vi "zigzag.vi"(4 "angulo":dbl=90.0 format="%#_13g", 6 "points 3":cluster{"x":dbl, "y":dbl}[](array[cluster])=[{"x"=0.0, "y"=0.0}, {"x"=1000.0, "y"=1000.0}, {"x"=-1000.0, "y"=1000.0}], 8 "output angle":dbl=4.0, 9 "output xy":dbl=2.0, 10 "Current Robot":T1={"id"=0, "function"=enum."Attacker", "x"=0.0, "y"=0.0, "orientation"=0.0, "v_tangent"=0.0, "v_normal"=0.0, "v_ang"=0.0, "kick_x"=0.0, "kick_z"=0.0, "dribble"=FALSE, "Timestamp"=timestamp(0 s since 1904-01-01), "dest_x"=0.0, "dest_y"=0.0, "dest_orientation"=0.0, "estimatives"={"est_v_tangent"=0.0, "est_v_normal"=0.0, "est_vx"=0.0, "est_vy"=0.0, "Pos Robot Est"=[]}, "dest_x_kick"=0.0, "dest_y_kick"=0.0, "Gap Coord"=[], "States"=enum."GoToTangent", "Path "=[], "Path  Smooth"=[], "dest_vel"=0.0}, 11 "Al Input":T4={"our_robots"=[], "enemy_robots"=[], "balls"=[], "geometry"={"line_width"=0, "field_length"=0, "field_width"=0, "boundary_width"=0, "referee_width"=0, "goal_width"=0, "goal_depth"=0, "goal_wall_width"=0, "center_circle_radius"=0, "defense_radius"=0, "defense_stretch"=0, "free_kick_from_defense_dist"=0, "penalty_spot_from_field_line_dist"=0, "penalty_line_from_spot_dist"=0}, "IA Judge"={"stage"="", "command"="", "our_goalie_id"=0.0, "enemy_goalie_id"=0.0, "command enum"=enum."Halt", "Time"=enum."Azul"}, "Received Timestamp"=timestamp(0 s since 1904-01-01), "Events"={"Touch"=FALSE, "Ball out"=FALSE, "id touch"=0.0, "Ball out of \nVision"=FALSE, "Ball inside \nGoalie area"=FALSE, "Robot not responding"=FALSE, "Robots responding status"=[1.0, 1.0, 1.0, 1.0, 1.0, 1.0], "Enemy Ball \nPossession"=FALSE, "Pass State"=FALSE, "id end of pass"=0.0, "Kick"=FALSE, "Id ini Possession"=0.0, "Ball Possesion"=FALSE, "Id Possesion"=0.0}}) -> (3 "Output Robot":T1={"id"=0, "function"=enum."Attacker", "x"=0.0, "y"=0.0, "orientation"=0.0, "v_tangent"=0.0, "v_normal"=0.0, "v_ang"=0.0, "kick_x"=0.0, "kick_z"=0.0, "dribble"=FALSE, "Timestamp"=timestamp(0 s since 1904-01-01), "dest_x"=0.0, "dest_y"=0.0, "dest_orientation"=0.0, "estimatives"={"est_v_tangent"=0.0, "est_v_normal"=0.0, "est_vx"=0.0, "est_vy"=0.0, "Pos Robot Est"=[]}, "dest_x_kick"=0.0, "dest_y_kick"=0.0, "Gap Coord"=[], "States"=enum."GoToTangent", "Path "=[], "Path  Smooth"=[], "dest_vel"=0.0})   [LabVIEW 2017]
uses:
  Core/AI Input.ctl
  Core/AI Robot.ctl
  Intel/Functions Enum.ctl
  Intel/AttackerStates.ctl
  Core/AI Ball.ctl
  Core/Field Size.ctl
  Core/AI Judge.ctl
  Intel/Command Enum.ctl
  Util/Events/Events.ctl
panel:
  out "Waveform Chart 3":dbl(graph)
  out "Waveform Chart 2":dbl(graph)
  out "Waveform Chart":dbl(graph)
  in  "polar tolerance":dbl=50.0 format="%#_13g"
  in  "?":bool=TRUE
  out "element 2":cluster{"x":dbl, "y":dbl}
  in  "square tolerance":dbl=50.0 format="%#_13g"
  # "polar check"
  # "cartesian check"
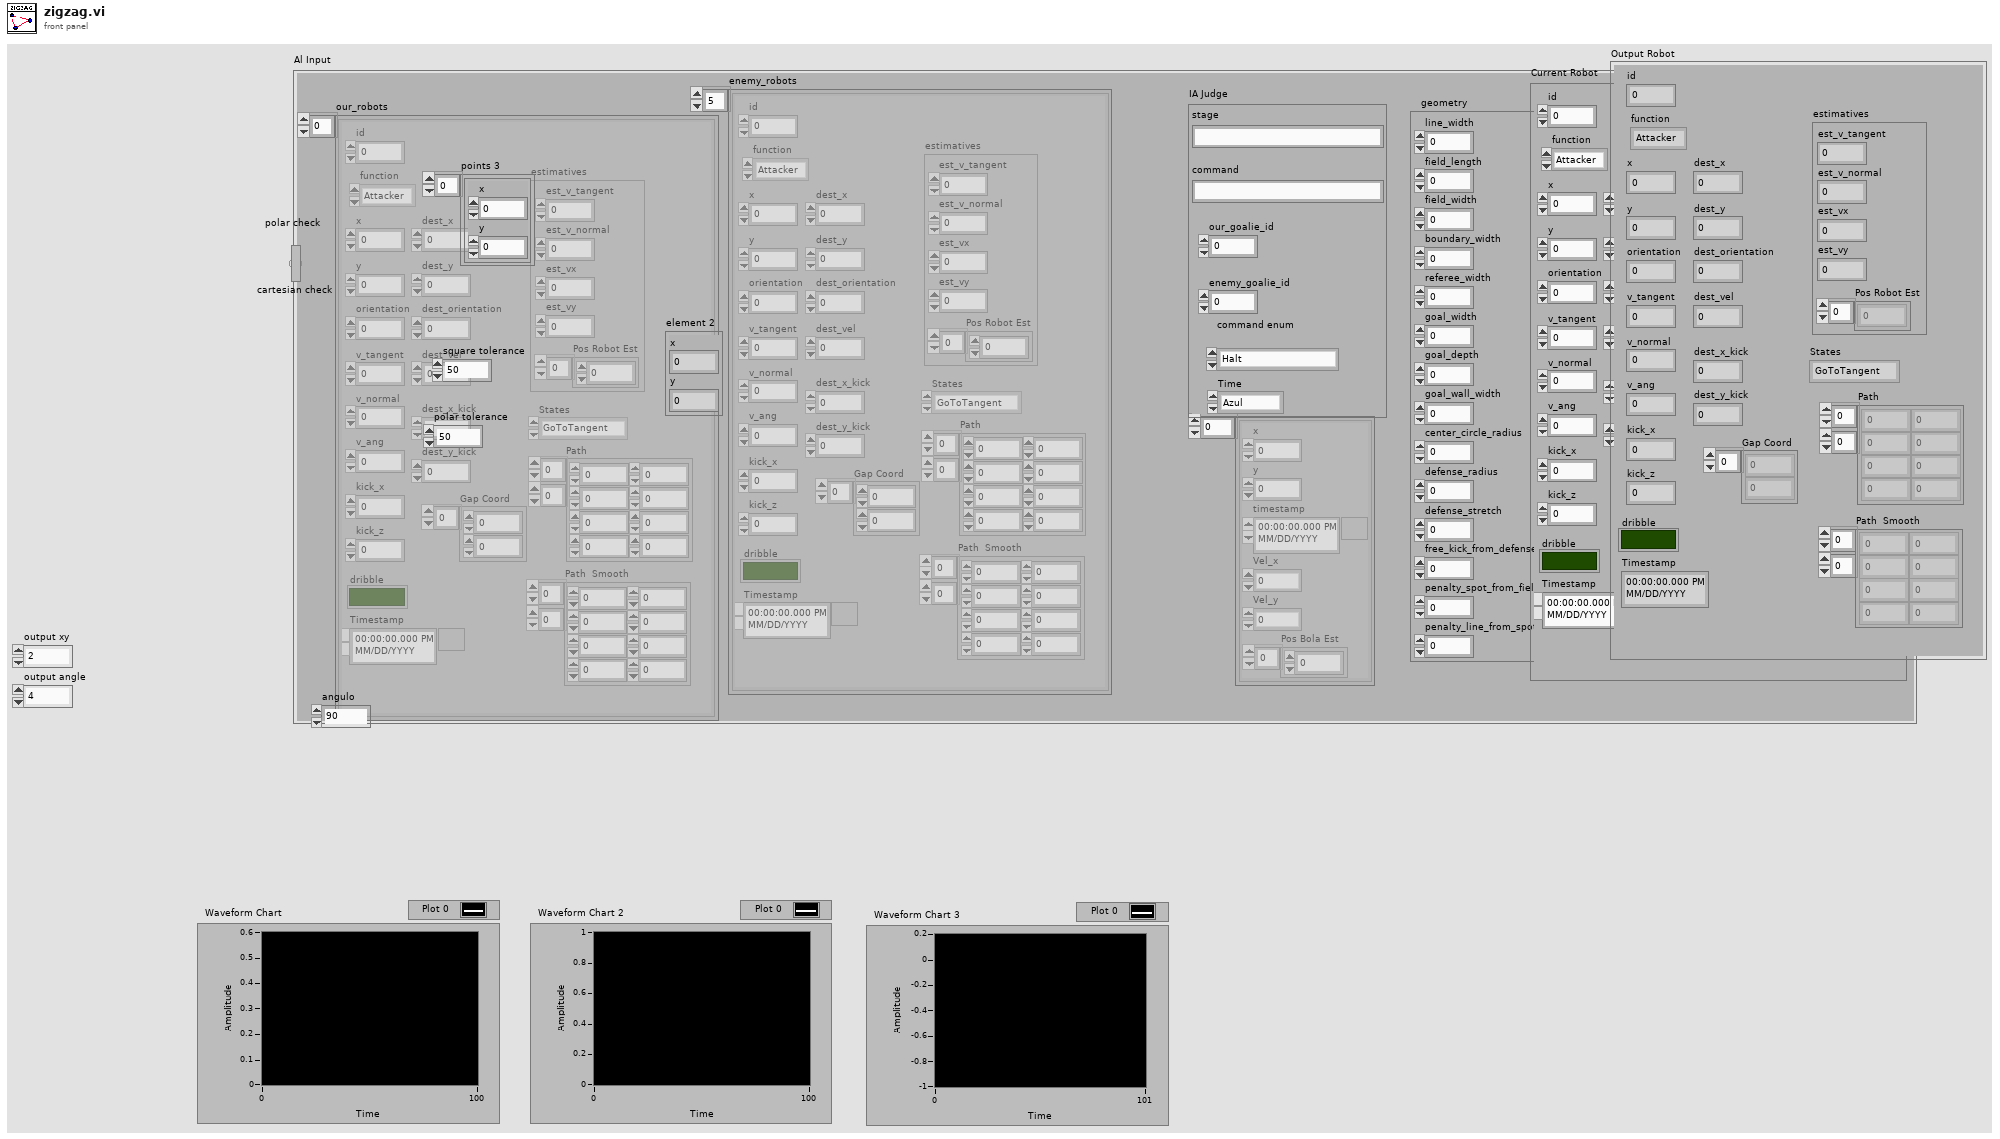
[diagram p1: front panel]
types:
  T1 = typedef "AI Robot.ctl" = cluster{"id":u32, "function":T2, "x":dbl, "y":dbl, "orientation":dbl, "v_tangent":dbl, "v_normal":dbl, "v_ang":dbl, "kick_x":dbl, "kick_z":dbl, "dribble":bool, "Timestamp":timestamp, "dest_x":dbl, "dest_y":dbl, "dest_orientation":dbl, "estimatives":cluster{"est_v_tangent":dbl, "est_v_normal":dbl, "est_vx":dbl, "est_vy":dbl, "Pos Robot Est":dbl[]}, "dest_x_kick":dbl, "dest_y_kick":dbl, "Gap Coord":dbl[], "States":T3, "Path ":dbl[][], "Path  Smooth":dbl[][], "dest_vel":dbl}
  T2 = typedef "Functions Enum.ctl" = enum16{"Attacker", "Goalie", "Defender", "Striker", "Goto 0", "Dummy", "Kicker", "ZigZag"}
  T3 = typedef "AttackerStates.ctl" = enum16{"Pass", "GoToTangent", "BallGetting", "GoToKick", ""}
  T4 = typedef "AI Input.ctl" = cluster{"our_robots":T1[], "enemy_robots":T1[], "balls":T5[], "geometry":T6, "IA Judge":T7, "Received Timestamp":timestamp, "Events":T9}
  T5 = typedef "AI Ball.ctl" = cluster{"x":dbl, "y":dbl, "timestamp":timestamp, "Vel_x":dbl, "Vel_y":dbl, "Pos Bola Est":dbl[]}
  T6 = typedef "Field Size.ctl" = cluster{"line_width":u32, "field_length":u32, "field_width":u32, "boundary_width":u32, "referee_width":u32, "goal_width":u32, "goal_depth":u32, "goal_wall_width":u32, "center_circle_radius":u32, "defense_radius":u32, "defense_stretch":u32, "free_kick_from_defense_dist":u32, "penalty_spot_from_field_line_dist":u32, "penalty_line_from_spot_dist":u32}
  T7 = typedef "AI Judge.ctl" = cluster{"stage":string, "command":string, "our_goalie_id":dbl, "enemy_goalie_id":dbl, "command enum":T8, "Time":enum16{"Azul", "Amarelo"}}
  T8 = typedef "Command Enum.ctl" = enum16{"Halt", "Stop", "Force Start", "PKA Normal Start", "Prepare Kickoff Ally", "PKE Normal Start", "Prepare Kickoff Enemy", "Prepare Penalty Ally", "PPA Normal Start", "Prepare Penalty Enemy", "PPE Normal Start", "Direct Free Enemy", "Direct Free Ally", "Indirect Free Enemy", "Indirect Free Ally", "Timeout Enemy", "Timeout Ally", "Goal Enemy", "Goal Ally", "Ball Placement Enemy", "Ball Placement Ally", "Normal Half Time", "Extra Time Break", "Extra Half Time", "None", "Post Game"}
  T9 = typedef "Events.ctl" = cluster{"Touch":bool, "Ball out":bool, "id touch":dbl, "Ball out of \nVision":bool, "Ball inside \nGoalie area":bool, "Robot not responding":bool, "Robots responding status":dbl[], "Enemy Ball \nPossession":bool, "Pass State":bool, "id end of pass":dbl, "Kick":bool, "Id ini Possession":dbl, "Ball Possesion":bool, "Id Possesion":dbl}
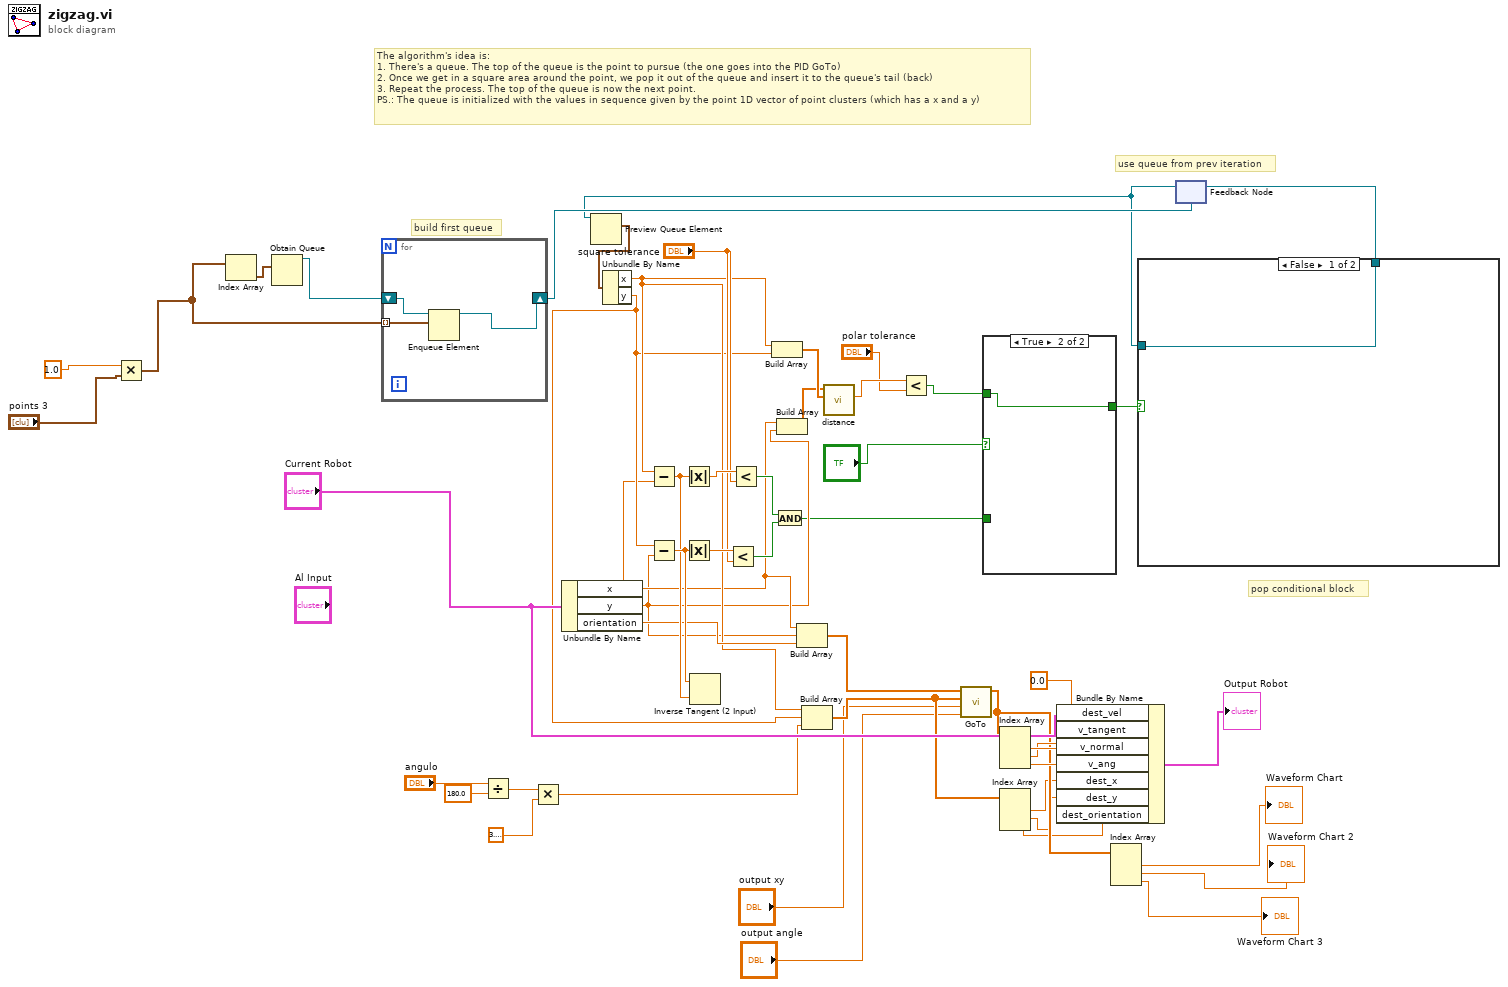
[diagram p0: block diagram]
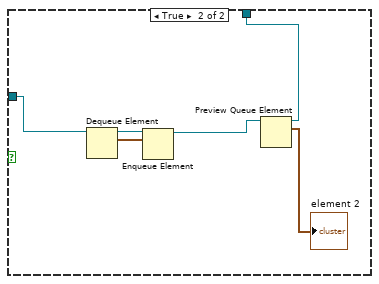
[diagram p3: hidden frame]
diagram:
  # "pop conditional block"
  # "use queue from prev iteration"
  # "The algorithm's idea is:\n1. There's a queue. The top of the queue is the point to pursue (the one goes into the PID GoTo)\n2. Once we get in a square area around the point, we pop it out of the queue and insert it to the queue's tail (back)\n3. Repeat the process. The top of the queue is now the next point.\nPS.: The queue is initialized with the values in sequence given by the point 1D vector of point clusters (which has a x and a y)"
  # "build first queue"
  n1 = Multiply(x=1.0, y="points 3") -> (x*y=w17:cluster{"x":dbl, "y":dbl}[])
  n2 = Index Array(array=w17) -> (element=w51:cluster{"x":dbl, "y":dbl})  [unwired: 1 in]
  n3 = Obtain Queue(element data type=w51) -> (queue out=w50:refnum<queue>)  [unwired: 4 in, 2 out]
  n4 = for {
    tunnel: w17 -> [w53] mode=indexing
    shift-right: [w54] -> w43
    shift-left: w50 -> [w52]
    n5 = Enqueue Element(queue=w52, element=w53) -> (queue out=w54:refnum<queue>)  [unwired: 2 in, 2 out]
  }
  n6 = Divide(x="angulo", y=180.0) -> (x/y=w4:dbl)
  n7 = Multiply(x=w4, y=3.141592653589793) -> (x*y=w2:dbl)
  n8 = Unbundle By Name("Current Robot") -> ("x"=w28:dbl, "y"=w27:dbl, "orientation"=w39:dbl)
  n9 = Build Array(w28, w27) -> (w26:dbl[])
  n10 = Build Array(w28, w27, w39) -> (w38:dbl[])
  n11 = feedback #1(w43) -> (w42:refnum<queue>)
  n12 = Preview Queue Element(queue=w42) -> (element=w49:cluster{"x":dbl, "y":dbl})  [unwired: 2 in, 3 out]
  n13 = Unbundle By Name(w49) -> ("x"=w31:dbl, "y"=w30:dbl)
  n14 = Subtract(x=w31, y=w28) -> (x-y=w40:dbl)
  n15 = Subtract(x=w30, y=w27) -> (x-y=w41:dbl)
  n16 = Absolute Value(x=w40) -> (abs(x)=w48:dbl)
  n17 = Absolute Value(x=w41) -> (abs(x)=w47:dbl)
  n18 = Inverse Tangent (2 Input)(1:w40, 2:w41) -> ()  [unwired: 1 out]
  n19 = Less?(x=w47, y="square tolerance") -> (x < y?=w44:bool)
  n20 = Less?(x=w48, y="square tolerance") -> (x < y?=w45:bool)
  n21 = Build Array(w31, w30) -> (w29:dbl[])
  n22 = And(x=w45, y=w44) -> (x .and. y?=w20:bool)
  n23 = Build Array(w31, w30, w2) -> (w12:dbl[])
  n24 = call "distance.vi"("target pos"=w29, "obj pos"=w26) -> ("sqrt(x)"=w24:dbl)  [unwired: 9 in]
  n25 = Less?(x=w24, y="polar tolerance") -> (x < y?=w22:bool)
  n26 = call "GoTo.vi"("output angle"="output angle", "output xy"="output xy", "Target"=w12, "Position"=w38) -> ("Output\nVelocity"=w16:dbl[])  [unwired: 6 in, 1 out]
  n27 = case shown="True" "?" {
    tunnel: w22 -> [_ w56]
    tunnel: [w55 w56] -> w21
    tunnel: w20 -> [w55 _]
    frame False {
    }
    frame True {
    }
  }
  n28 = Index Array(array=w16) -> (element #1=w36:dbl, element #2=w35:dbl, element #3=w34:dbl)  [unwired: 3 in]
  n29 = Index Array(array=w12) -> (element #1=w11:dbl, element #2=w10:dbl, element #3=w9:dbl)  [unwired: 3 in]
  n30 = Bundle By Name(cluster="Current Robot", "dest_vel"=0.0, "v_tangent"=w36, "v_normal"=w35, "v_ang"=w34, "dest_x"=w11, "dest_y"=w10, "dest_orientation"=w9) -> (→"Output Robot":T1)
  n31 = Index Array(array=w16) -> (element #1=→"Waveform Chart":dbl, element #2=→"Waveform Chart 2":dbl, element #3=→"Waveform Chart 3":dbl)  [unwired: 3 in]
  n32 = case shown="False" w21 {
    tunnel: w42 -> [w57 w61]
    tunnel: [w57 w58] -> w32
    frame False {
    }
    frame True {
      n33 = Dequeue Element(queue=w61) -> (queue out=w62:refnum<queue>, element=w63:cluster{"x":dbl, "y":dbl})  [unwired: 2 in, 2 out]
      n34 = Enqueue Element(queue=w62, element=w63) -> (queue out=w60:refnum<queue>)  [unwired: 2 in, 2 out]
      n35 = Preview Queue Element(queue=w60) -> (queue out=w58:refnum<queue>, element=→"element 2":cluster{"x":dbl, "y":dbl})  [unwired: 2 in, 2 out]
    }
  }
  n36 = feedback-in #1(w32) -> ()
